vi "init_TRIG1.vi"(7 "reset":bool, 11 "VISA resource name":refnum<visa-resource-name>) -> (0 "error out":errorcluster, 3 "VISA resource name out":refnum<visa-resource-name>)   [LabVIEW 2012]
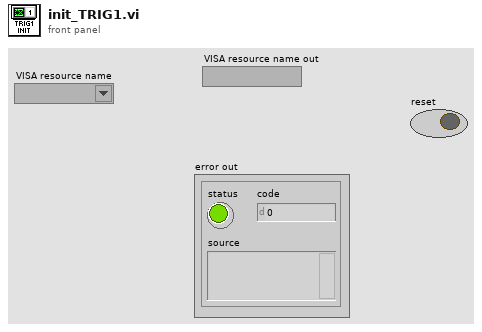
[diagram p1: front panel]
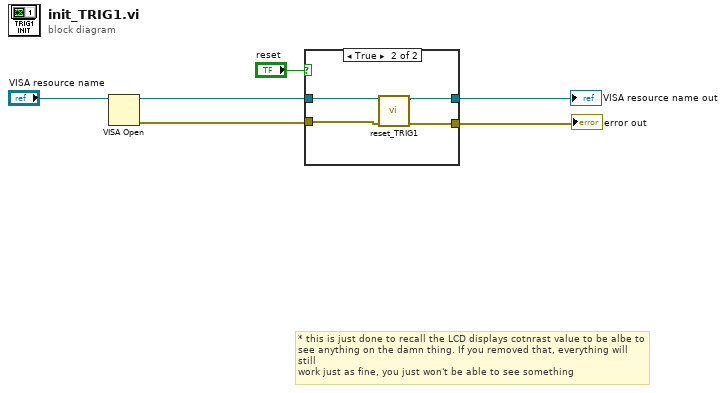
[diagram p0: block diagram]
diagram:
  # "* this is just done to recall the LCD displays cotnrast value to be albe to \nsee anything on the damn thing. If you removed that, everything will still\nwork just as fine, you just won't be able to see something"
  n1 = VISA Open(VISA resource name="VISA resource name") -> (VISA resource name=w2:refnum<visa-resource-name>, error out=w1:errorcluster)  [unwired: 4 in]
  n2 = case shown="True" "reset" {
    tunnel: w2 -> [w8 w12]
    tunnel: [w8 w11] -> w5
    tunnel: w1 -> [w7 w10]
    tunnel: [w7 w9] -> w4
    frame False {
    }
    frame True {
      n3 = call "reset_TRIG1.vi"("error in (no error)"=w10, "VISA resource name"=w12) -> ("error out"=w9:errorcluster, "VISA resource name out"=w11:refnum<visa-resource-name>)  [unwired: 8 in]
    }
  }
  "VISA resource name out" <- w5
  "error out" <- w4
